vi "Tektronix DPO MSO 2000 4000 Series Edge Triggered Acquisition Waveform Example.vi"() -> ()   [LabVIEW 2017]
doc: "This example VI illustrates how to configure an oscilloscope to generate an edge trigger and acquire a waveform from that trigger using the following steps:\n\n1. Specify a valid VISA session. \n2. Specify a channel. \n3. Specify a vertical offset, range, and coupling method for the channel you selected. \n4. Specify the acquisition type. \n5. Specify the timebase and record length. \n6. Specify the trigger level for the edge trigger. \n7. Run the VI. The graph displays the waveform you acquire."
uses:
  <instrlib>/Tektronix DPO MSO 2000 4000 Series/Public/Configure/Configure Trigger (Edge).vi
  <instrlib>/Tektronix DPO MSO 2000 4000 Series/Tektronix DPO MSO 2000 4000 Series.lvlib
panel:
  in  "Record Length (10: 10k points)":u32(ring)=10 items=["1000 points"=1, "10k points"=10, "100k points"=100, "1M points"=1000, "10M points"=10000]
  in  "Maximum Time (10000ms)":u32=10000
  in  "Vertical Coupling (1: DC)":u16(ring)=1 items=["AC", "DC", "Ground"]
  in  "VISA Resource Name":refnum<visa-resource-name>
  in  "Channel (0: Channel 1)":u16(ring) items=["Channel 1", "Channel 2", "Channel 3", "Channel 4", "Math", "Reference 1", "Reference 2", "Reference 3", "Reference 4"]
  in  "Trigger Level (0.0)":dbl
  in  "Timebase (4.0e-5)":dbl=4e-05
  in  "Vertical Range (1.0)":dbl=1.0
  in  "Vertical Offset (0)":dbl
  out "Waveform Graph":waveform(dbl)(graph)
  # "(C) 2006 - 2016. National Instruments Corporation. ALL RIGHTS RESERVED."
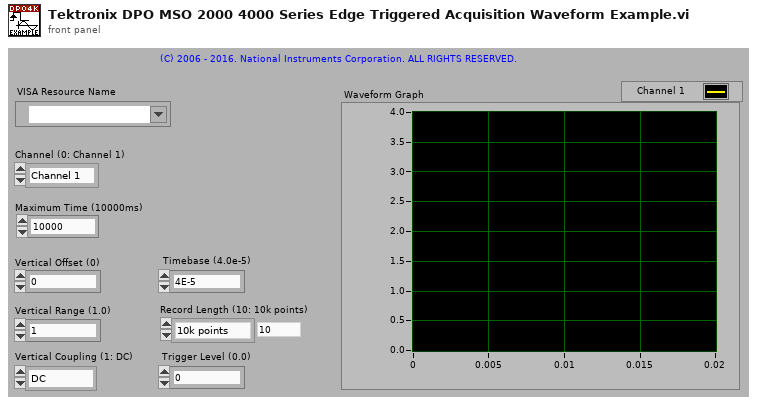
[diagram p1: front panel]
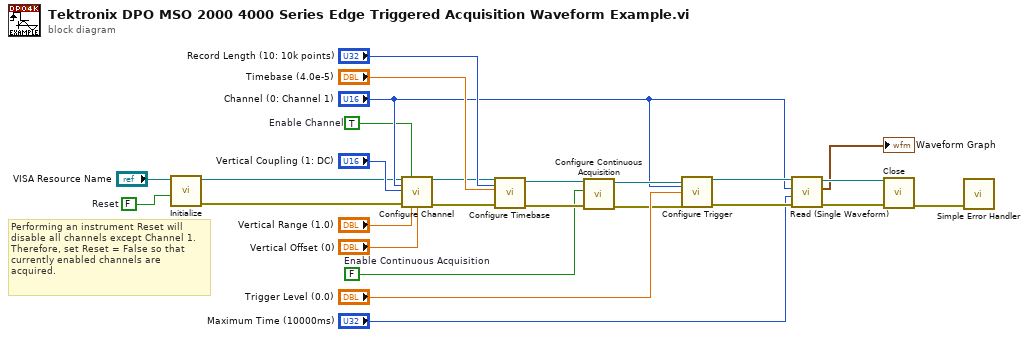
[diagram p0: block diagram]
diagram:
  w9 = FALSE  # Enable Continuous Acquisition
  w3 = TRUE  # Enable Channel
  w14 = FALSE  # Reset
  # "Performing an instrument Reset will disable all channels except Channel 1. Therefore, set Reset = False so that currently enabled channels are acquired."
  n1 = call <instrlib>:"Initialize.vi"("Reset (True)"=w14, "VISA resource name"="VISA Resource Name") -> ("error out"=w4:errorcluster, "VISA resource name out"=w5:refnum<visa-resource-name>)  [unwired: 8 in]
  n2 = call <instrlib>:"Configure Channel.vi"("VISA resource name"=w5, "Enable Channel (T: Enable)"=w3, "Channel (0: Channel 1)"="Channel (0: Channel 1)", "Vertical Coupling (1: DC)"="Vertical Coupling (1: DC)", "error in (no error)"=w4, "Vertical Range (10.0 V)"="Vertical Range (1.0)", "Vertical Offset (0.0 V)"="Vertical Offset (0)") -> ("VISA resource name out"=w13:refnum<visa-resource-name>, "error out"=w12:errorcluster)  [unwired: 7 in]
  n3 = call <instrlib>:"Configure Timebase.vi"("Record Length (10: 10k points)"="Record Length (10: 10k points)", "error in (no error)"=w12, "Timebase (0.0005 s)"="Timebase (4.0e-5)", "VISA resource name"=w13) -> ("error out"=w10:errorcluster, "VISA resource name out"=w11:refnum<visa-resource-name>)  [unwired: 6 in]
  n4 = call <instrlib>:"Configure Continuous Acquisition.vi"("error in (no error)"=w10, "Enable Continuous Acquisition Mode (T: Enable)"=w9, "VISA resource name"=w11) -> ("error out"=w7:errorcluster, "VISA resource name out"=w8:refnum<visa-resource-name>)  [unwired: 7 in]
  n5 = call-poly <instrlib>:"Configure Trigger.vi"("VISA resource name"=w8, "Trigger Source (0: Channel 1)"="Channel (0: Channel 1)", "Trigger Level (0.0 V)"="Trigger Level (0.0)", "error in (no error)"=w7) -> ("VISA resource name out"=w23:refnum<visa-resource-name>, "error out"=w18:errorcluster)  [unwired: 10 in]
  n6 = call <instrlib>:"Read (Single Waveform).vi"("error in (no error)"=w18, "Maximum Time (10000ms)"="Maximum Time (10000ms)", "Channel (0: Channel 1)"="Channel (0: Channel 1)", "VISA resource name"=w23) -> ("error out"=w17:errorcluster, "Waveform Graph"=→"Waveform Graph":waveform(dbl), "VISA resource name out"=w21:refnum<visa-resource-name>)  [unwired: 5 in]
  n7 = call <instrlib>:"Close.vi"("error in (no error)"=w17, "VISA resource name"=w21) -> ("error out"=w22:errorcluster)  [unwired: 9 in]
  n8 = call <vilib>:"Simple Error Handler.vi"("error in (no error)"=w22) -> ()  [unwired: 4 in, 5 out]
